vi "Min_Max.vi"() -> ()   [LabVIEW 2019]
panel:
  out "min(x,y)":dbl
  out "max(x,y)":dbl
  in  "Numeric 2":dbl
  in  "Numeric":dbl
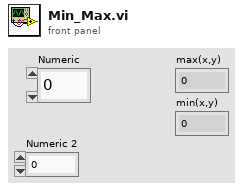
[diagram p1: front panel]
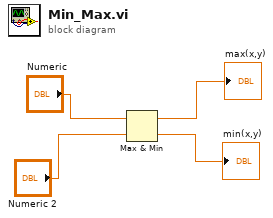
[diagram p0: block diagram]
diagram:
  n1 = Max & Min(x="Numeric", y="Numeric 2") -> (max(x,y)=→"max(x,y)":dbl, min(x,y)=→"min(x,y)":dbl)
